vi "rvc 2D Homogeneous to Euler 2.vi"(8 "error in (no error)":errorcluster, 11 "T":dbl[][](array[numeric])) -> (0 "Error Out":errorcluster, 1 "y":dbl, 2 "x":dbl, 3 "Array":dbl[](array[numeric]), 4 "z":dbl)   [LabVIEW 2014]
uses:
  <vilib>/Utility/error.llb/Error Cluster From Error Code.vi
  <vilib>/ErrorRing/Error Ring.xnode
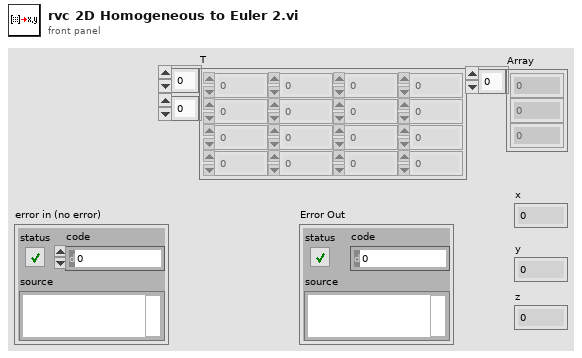
[diagram p1: front panel]
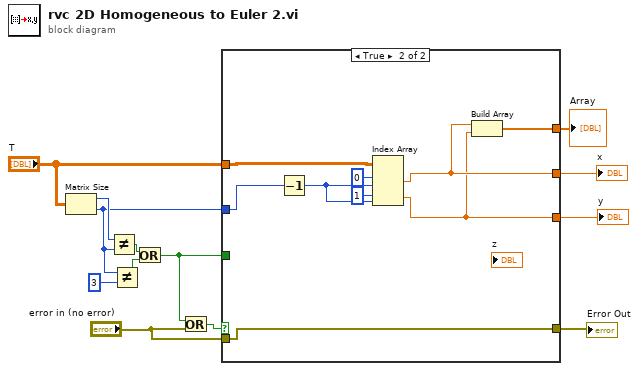
[diagram p0: block diagram]
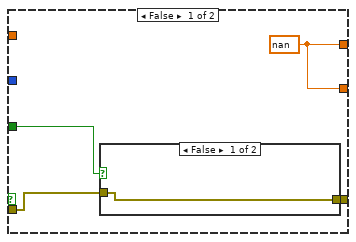
[diagram p2: hidden frame]
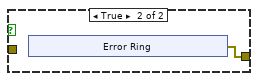
[diagram p3: hidden frame]
diagram:
  n1 = Matrix Size(0:"T") -> (1:w9:i32, 2:w6:i32)
  n2 = Not Equal?(x=w9, y=w6) -> (x != y?=w8:bool)
  n3 = Not Equal?(x=w6, y=3) -> (x != y?=w7:bool)
  n4 = Or(x=w8, y=w7) -> (x .or. y?=w2:bool)
  n5 = Or(x=w2, y="error in (no error)") -> (x .or. y?=w4:bool)
  n6 = case shown="True" w4 {
    tunnel: [w14 w30] -> w13
    tunnel: "T" -> [_ w28]
    tunnel: w6 -> [_ w32]
    tunnel: [w17 w26] -> w11
    tunnel: [w17 w25] -> w10
    tunnel: "error in (no error)" -> [w15 w30]
    tunnel: w2 -> [w16 _]
    tunnel: [_ w24] -> w1
    frame False {
      w17 = nan ("x")
      n7 = case shown="False" w16 {
        tunnel: w15 -> [w18 _]
        tunnel: [w18 w19] -> w14
        frame False {
        }
        frame True {
          n8 = xnode "Error Ring"() -> ("error out"=w19:errorcluster)
        }
      }
    }
    frame True {
      n9 = Decrement(x=w32) -> (x-1=w27:i32)
      n10 = Index Array(array=w28, index (row) #1=0 ("disabled index (row)"), index (col) #1=w27, index (row) #2=1 ("disabled index (row)"), index (col) #2=w27) -> (element #1=w26:dbl, element #2=w25:dbl)
      n11 = Build Array(w26, w25) -> (w24:dbl[])
    }
  }
  "x" <- w11
  "y" <- w10
  "Error Out" <- w13
  "Array" <- w1
